vi "ACCEL_TEST_R2.vi"() -> ()   [LabVIEW 2015]
uses:
  <vilib>/myRIO/Instrument Drivers/Onboard Devices/Accelerometer/typedefs/Accelerometer Reference.ctl
  <vilib>/myRIO/Common/Instrument Driver Framework/Utilities/typedefs/myRIO Generic Hardware Reference.ctl
  <vilib>/myRIO/Common/Instrument Driver Framework/Utilities/typedefs/Hardware Version Enum.ctl
  <vilib>/myRIO/Common/Instrument Driver Framework/Utilities/typedefs/myRIO v1.0 Reference.ctl
  <vilib>/myRIO/Common/Instrument Driver Framework/Utilities/typedefs/Generic FPGA Reference.ctl
  <vilib>/myRIO/Common/Instrument Driver Framework/myRIO v1.0/Accelerometer/typedefs/Accelerometer Channels List.ctl
  <vilib>/myRIO/Common/Instrument Driver Framework/myRIO v1.0/Accelerometer/typedefs/Accelerometer Channels Enum.ctl
  <vilib>/userdefined/High Color/nirio_resource_hc.ctl
  <vilib>/myRIO/Common/Instrument Driver Framework/Utilities/vis/Is FPGA Ref Available.vi
  <vilib>/myRIO/Common/Instrument Driver Framework/myRIO v1.0/Accelerometer/vis/myRIO v1.1 Open Accelerometer.vi
  <vilib>/myRIO/Instrument Drivers/Onboard Devices/Accelerometer/vis/Read.vi
  <vilib>/Analysis/8numeric.llb/1D Numeric Integration.vi
  <vilib>/myRIO/Common/Instrument Driver Framework/Utilities/vis/Validate Channels.vi
  <vilib>/myRIO/Common/Instrument Driver Framework/myRIO v1.0/Accelerometer/vis/myRIO v1.0 Reserve Accelerometer.vi
  <vilib>/myRIO/Common/Instrument Driver Framework/myRIO v1.0/Resource Manager/vis/myRIO v1.0 Reserve Channel List.vi
  <vilib>/myRIO/Common/Instrument Driver Framework/myRIO v1.0/Accelerometer/vis/myRIO v1.0 Build MUX Configuration Accelerometer.vi
  <vilib>/myRIO/Common/Instrument Driver Framework/myRIO v1.0/Resource Manager/vis/myRIO v1.0 Reserve Channel.vi
  <vilib>/myRIO/Common/Instrument Driver Framework/myRIO v1.0/Resource Manager/vis/myRIO v1.0 Unreserve Channel.vi
  <vilib>/myRIO/Common/Instrument Driver Framework/myRIO v1.0/Resource Manager/vis/myRIO v1.0 Build Mutex Name.vi
  <vilib>/Utility/VariantDataType/GetNumericInfo.vi
  <vilib>/Utility/error.llb/Error Cluster From Error Code.vi
  <vilib>/myRIO/Common/Instrument Driver Framework/myRIO v1.0/myRIO v1.1 Open.vi
  <vilib>/myRIO/Common/Instrument Driver Framework/myRIO v1.0/Accelerometer/vis/myRIO v1.0 Get Scaling Constant Accelerometer.vi
  <vilib>/myRIO/Common/Instrument Driver Framework/Utilities/vis/IO Manager.vi
  <vilib>/myRIO/Common/Instrument Driver Framework/Utilities/vis/Configuration Manager.vi
  <vilib>/myRIO/Common/Instrument Driver Framework/myRIO v1.0/myRIO v1.0 Close.vi
  <vilib>/myRIO/Common/Instrument Driver Framework/myRIO v1.0/Accelerometer/vis/myRIO v1.0 Read Accelerometer.vi
  <vilib>/myRIO/Express VI/Onboard Devices/Accelerometer/Accelerometer Express VI.xnode
  <vilib>/myRIO/Instrument Drivers/Onboard Devices/Accelerometer/vis/myRIO Accelerometer Open.xnode
  <vilib>/myRIO/Instrument Drivers/Onboard Devices/Accelerometer/Accelerometer.lvlib
  <vilib>/Analysis/NI_AALPro.lvlib
panel:
  in  "Min Threshold (X axis)":dbl=0.15 format="%#_13g"
  out "Velocity":dbl(graph)
  in  "Min delta Position":dbl=0.05 format="%#_13g"
  in  "stop":bool
  out "X-Axis (smoothed)":dbl
  out "Waveform Chart X":dbl(graph)
  out "Position":dbl(graph)
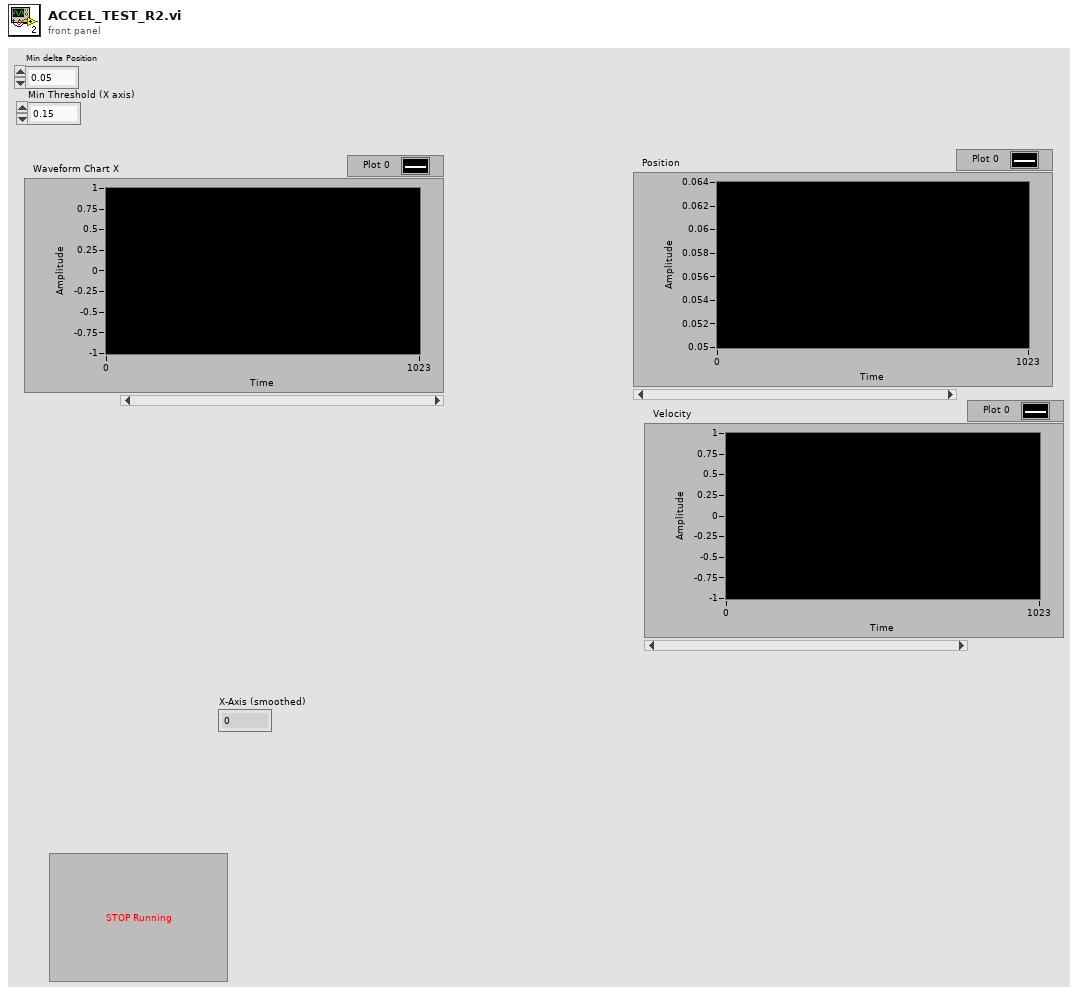
[diagram p1: front panel]
types:
  T1 = typedef "Accelerometer.lvlib/Accelerometer Reference.ctl" = cluster{"myRIO Reference":T2, "Accelerometer Channels List":T6, "LSB Weight":dbl}
  T2 = typedef "myRIO Generic Hardware Reference.ctl" = cluster{"myRIO Model":T3, "myRIO Hardware Reference":T4}
  T3 = typedef "Hardware Version Enum.ctl" = enum16{"Unknown", "myRIO-1900", "myRIO-1950", "roboRIO"}
  T4 = typedef "myRIO v1.0 Reference.ctl" = cluster{"Generic FPGA Reference":T5, "Allow multiple opens":bool}
  T5 = typedef "Generic FPGA Reference.ctl" = refnum<k20>
  T6 = typedef "Accelerometer Channels List.ctl" = T7[]
  T7 = typedef "Accelerometer Channels Enum.ctl" = enum16{"Not Connected", "X-Axis", "Y-Axis", "Z-Axis"}
  T8 = typedef "nirio_resource_hc.ctl" = tag
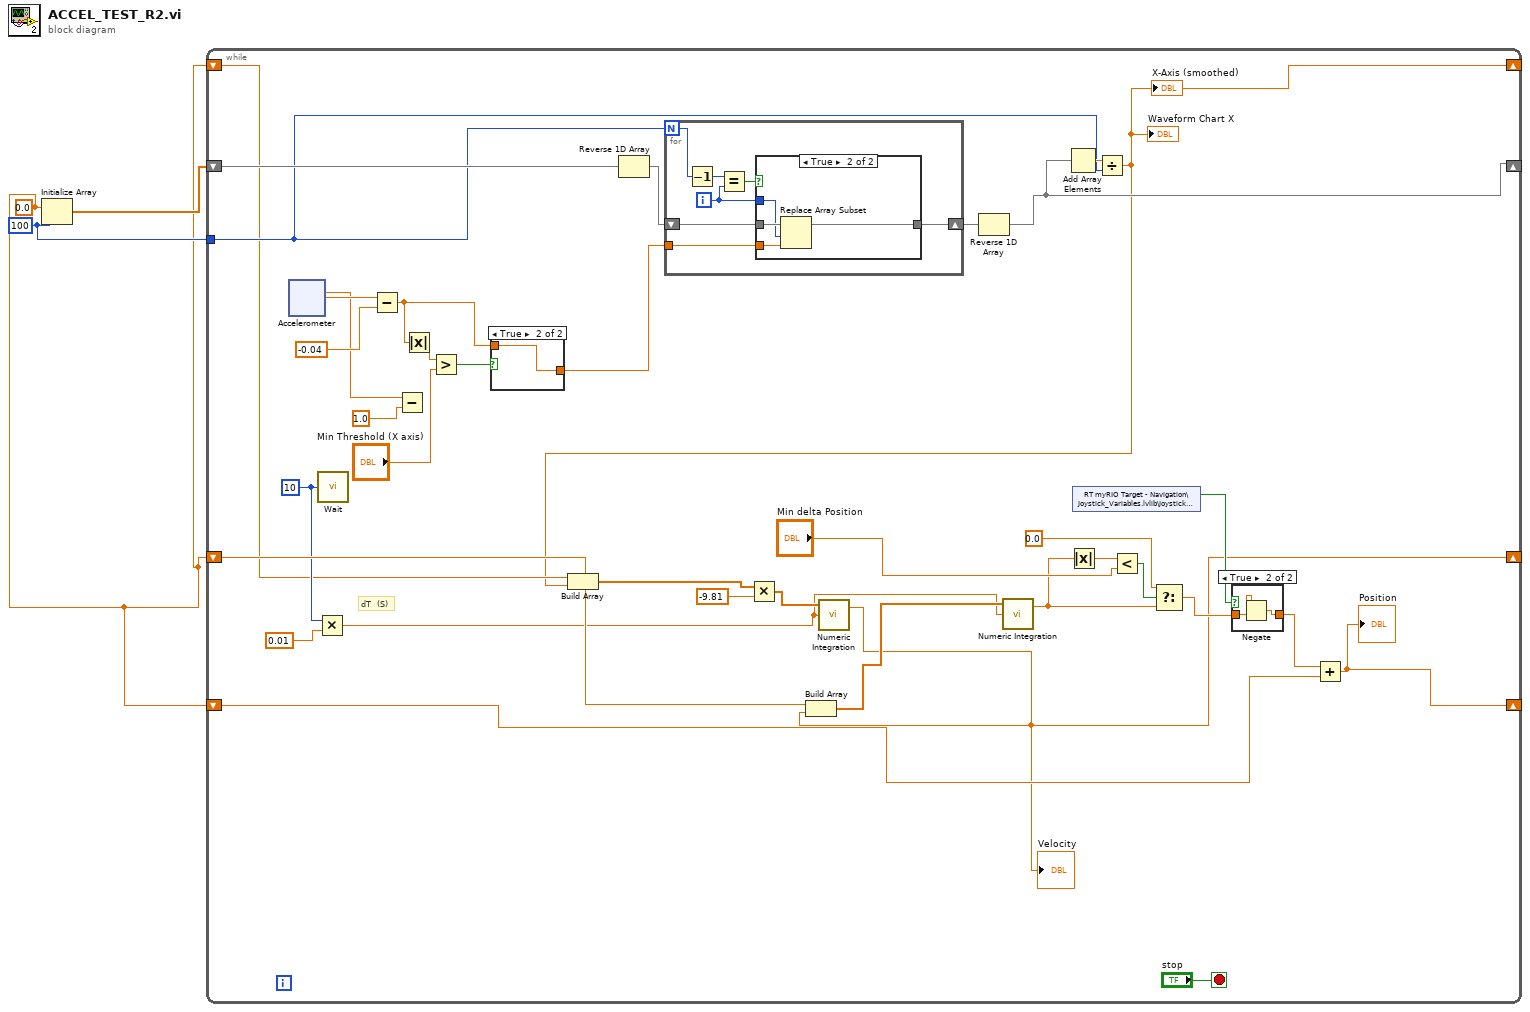
[diagram p0: block diagram]
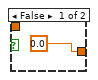
[diagram p3: hidden frame]
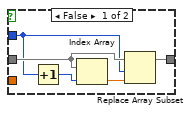
[diagram p4: hidden frame]
diagram:
  w3 = 100 ("dimension size")
  w1 = 0.0 ("element")
  n1 = Initialize Array(w1, w3) -> (w2:dbl[])
  n2 = while {
    shift-right: [w22] -> _
    shift-left: w2 -> [w36]
    tunnel: w3 -> [w24]
    shift-right: [w19] -> _
    shift-left: w1 -> [w23]
    shift-right: [w9] -> _
    shift-left: w1 -> [w32]
    shift-right: [w17] -> _
    shift-left: w1 -> [w18]
    stop <- "stop" stop-if-true
    w29 = u32 10 ("Count(mSec)")
    # "dT  (S)"
    n3 = xnode "Accelerometer"() -> ("X-Axis"=w20:dbl, "Y-Axis"=w7:dbl)  [unwired: 1 in, 1 out]
    n4 = Multiply(x=w29, y=0.01 ("element")) -> (x*y=w10:dbl)
    n5 = call "Wait"("Count(mSec)"=w29) -> ()  [unwired: 1 out]
    n6 = Subtract(x=w20, y=-0.04) -> (x-y=w25:dbl)
    n7 = Subtract(x=w7, y=1.0) -> ()  [unwired: 1 out]
    n8 = Absolute Value(x=w25) -> (abs(x)=w28:dbl)
    n9 = Greater?(x=w28, y="Min Threshold (X axis)") -> (0:w27:bool)
    n10 = case shown="True" w27 {
      tunnel: [0.0 ("y") w45] -> w21
      tunnel: w25 -> [_ w45]
      frame False {
      }
      frame True {
      }
    }
    n11 = Reverse 1D Array(array=w36) -> (reversed array=w39:dbl[])
    n12 = for {
      N: w24 -> [w51]
      shift-right: [w52] -> w38
      shift-left: w39 -> [w47]
      tunnel: w21 -> [w46]
      i -> [w48]
      n13 = Decrement(x=w51) -> (x-1=w49:i32)
      n14 = Equal?(x=w49, y=w48) -> (x = y?=w50:bool)
      n15 = case shown="True" w50 {
        tunnel: w48 -> [w54 w59]
        tunnel: w47 -> [w57 w60]
        tunnel: [w55 w61] -> w52
        tunnel: w46 -> [_ w58]
        frame False {
          n16 = Increment(x=w54) -> (x+1=w53:i32)
          n17 = Index Array(array=w57, index=w53) -> (element=w56:dbl)
          n18 = Replace Array Subset(array=w57, new element=w56, index=w54) -> (w55:dbl[])
        }
        frame True {
          n19 = Replace Array Subset(array=w60, new element=w58, index=w59) -> (w61:dbl[])
        }
      }
    }
    n20 = Reverse 1D Array(array=w38) -> (reversed array=w22:dbl[])
    n21 = Add Array Elements(numeric array=w22) -> (sum=w37:dbl)
    n22 = shared-variable "RT myRIO Target - Navigation\\Joystick_Variables.lvlib\\Joystick Direction"() -> (w16:bool)  [unwired: 1 in, 1 out]
    n23 = Divide(x=w37, y=w24) -> (x/y=w19:dbl)
    "X-Axis (smoothed)" <- w19
    "Waveform Chart X" <- w19
    n24 = Build Array(w23, w19) -> (w33:dbl[])
    n25 = Multiply(x=w33, y=-9.81 ("element")) -> (x*y=w34:dbl[])
    n26 = call-poly <vilib>:"Numeric Integration.vi"("dt"=w10, "Input Array"=w34) -> ("result"=w9:dbl)  [unwired: 1 in, 1 out]
    "Velocity" <- w9
    n27 = Build Array(w32, w9) -> (w31:dbl[])
    n28 = call-poly <vilib>:"Numeric Integration.vi"("dt"=w10, "Input Array"=w31) -> ("result"=w5:dbl)  [unwired: 1 in, 1 out]
    n29 = Absolute Value(x=w5) -> (abs(x)=w4:dbl)
    n30 = Less?(x=w4, y="Min delta Position") -> (x < y?=w13:bool)
    n31 = Select(t=0.0, s=w13, f=w5) -> (s? t:f=w11:dbl)
    n32 = case shown="True" w16 {
      tunnel: [w41 w42] -> w15
      tunnel: w11 -> [w41 w43]
      frame False {
      }
      frame True {
        n33 = Negate(x=w43) -> (-x=w42:dbl)
      }
    }
    n34 = Add(x=w15, y=w18) -> (x+y=w17:dbl)
    "Position" <- w17
  }
